vi "LS340_HeaterOutput.vi"(0 "VISA resource name":refnum<visa-resource-name>, 11 "error in (no error)":errorcluster) -> (4 "VISA resource name out":refnum<visa-resource-name>, 8 "Heater Output":dbl min=0.0 max=100.0 step=0.01 format="%.2f", 15 "error out":errorcluster)   [LabVIEW 2012]
doc: "This VI querys the instrument for the heater output in percent."
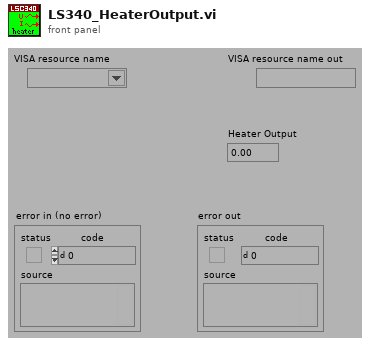
[diagram p1: front panel]
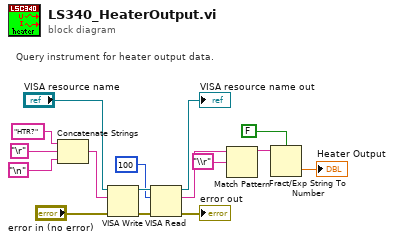
[diagram p0: block diagram]
diagram:
  # "Query instrument for heater output data."
  n1 = Concatenate Strings("HTR?", "\r", "\n") -> (w1:string)
  n2 = VISA Write(VISA resource name="VISA resource name", write buffer=w1, error in (no error)="error in (no error)") -> (VISA resource name out=w15:refnum<visa-resource-name>, error out=w14:errorcluster)  [unwired: 1 out]
  n3 = VISA Read(VISA resource name=w15, byte count=100, error in (no error)=w14) -> (VISA resource name out=→"VISA resource name out":refnum<visa-resource-name>, read buffer=w12:string, error out=→"error out":errorcluster)  [unwired: 1 out]
  n4 = Match Pattern(string=w12, regular expression="\\r") -> (before substring=w10:string)  [unwired: 1 in, 3 out]
  n5 = Fract/Exp String To Number(use system decimal point (T)=FALSE, string=w10) -> (number=→"Heater Output":dbl)  [unwired: 2 in, 1 out]
